vi "feedback.vi"() -> ()   [LabVIEW 2014]
panel:
  in  "닫기":bool
  in  "전송":bool
  in  "Subject":string="제목" caption="제목"
  in  "Message":string="제목을 입력해 주세요." caption="메시지"
  # "개발자에게 피드백"
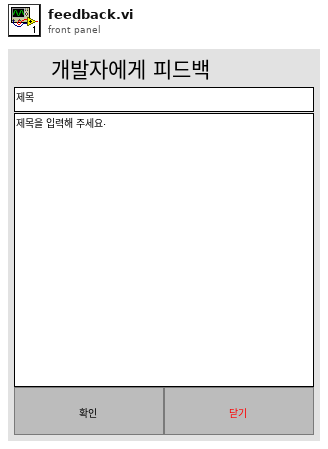
[diagram p1: front panel]
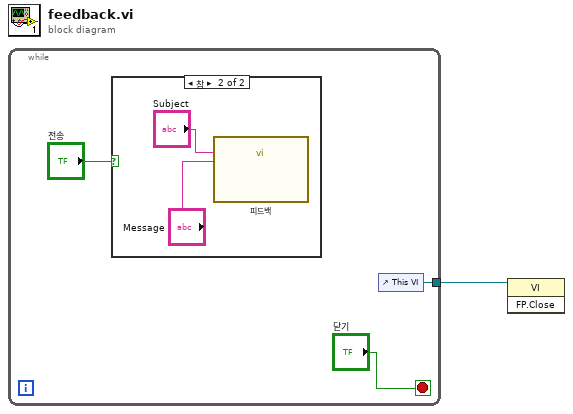
[diagram p0: block diagram]
diagram:
  n1 = while {
    tunnel: [w4] -> w1
    stop <- "닫기" stop-if-true
    n2 = case shown="참" "전송" {
      frame False {
      }
      frame True {
        n3 = call "피드백"("Message"="Message", "Subject"="Subject") -> ()  [unwired: 9 in, 1 out]
      }
    }
    n4 = control-ref of="This VI"() -> (w4:refnum<vi>)
  }
  n5 = invoke class="VI" method="FP.Close"(reference=w1) -> ()  [unwired: 2 in, 3 out]
